vi "init_avg_scope_Qs.vi"(2 "max summed queue size (-1, unlimited)":i32) -> (8 "avg_Q_data":T1)   [LabVIEW 2023]
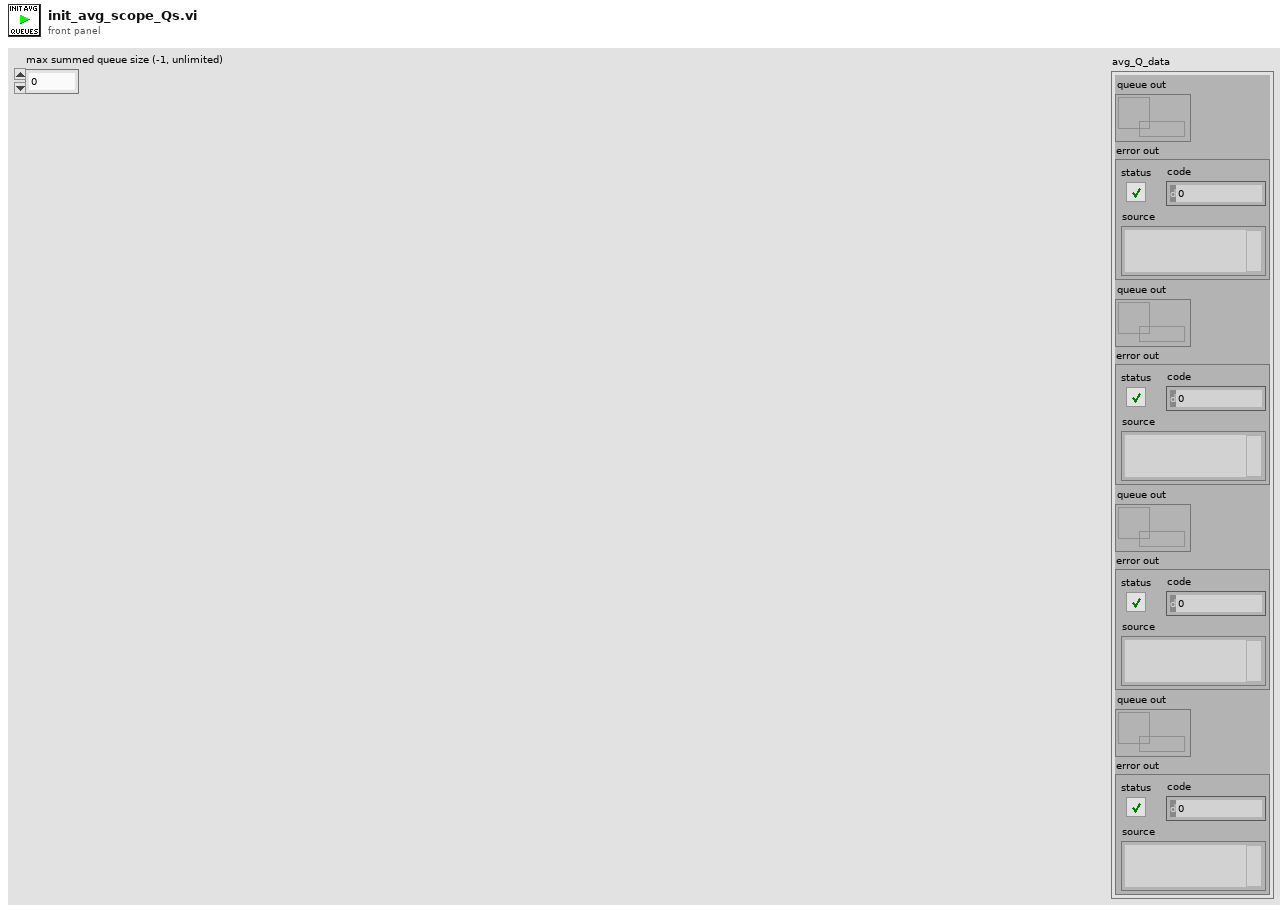
[diagram p1: front panel]
types:
  T1 = cluster{"queue out":refnum<queue>, "error out":errorcluster, "queue out":refnum<queue>, "error out":errorcluster, "queue out":refnum<queue>, "error out":errorcluster, "queue out":refnum<queue>, "error out":errorcluster}
  T2 = cluster{"wfm info":cluster{"actualSamples":i32, "absoluteInitialX":dbl, "relativeInitialX":dbl, "xIncrement":dbl, "offset":dbl, "gain":dbl, "reserved1":dbl, "reserved2":dbl}, "Offset WFm":waveform(dbl), bool}
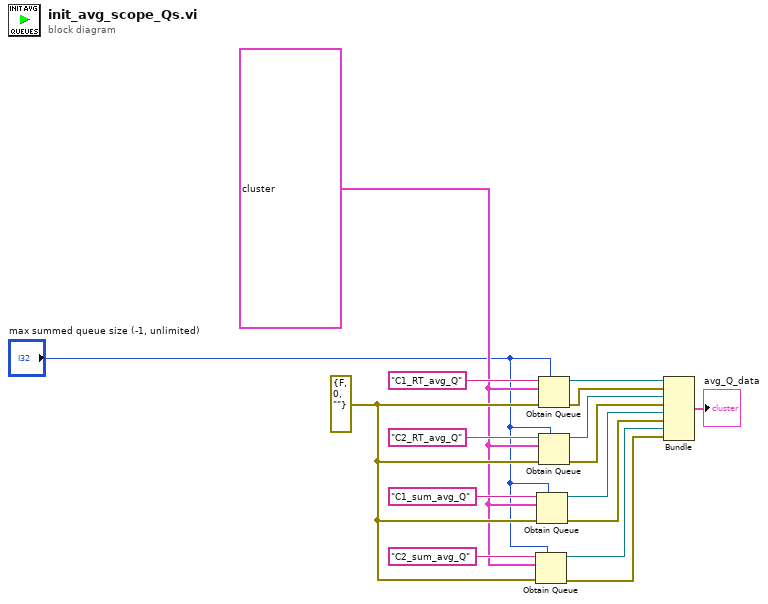
[diagram p0: block diagram]
diagram:
  w3 = T2 {"wfm info"={"actualSamples"=0, "absoluteInitialX"=0.0, "relativeInitialX"=0.0, "xIncrement"=0.0, "offset"=0.0, "gain"=0.0, "reserved1"=0.0, "reserved2"=0.0}, "Offset WFm"={"t0"=timestamp(0 s since 1904-01-01), "dt"=1.0, "Y"=[]}, FALSE} ("output cluster")
  w16 = errorcluster {"status"=FALSE, "code"=0, "source"=""} ("error in (no error)")
  n1 = Obtain Queue(max queue size (-1, unlimited)="max summed queue size (-1, unlimited)", name (unnamed)="C2_sum_avg_Q", element data type=w3, error in (no error)=w16) -> (queue out=w5:refnum<queue>, error out=w4:errorcluster)  [unwired: 1 in, 1 out]
  n2 = Obtain Queue(max queue size (-1, unlimited)="max summed queue size (-1, unlimited)", name (unnamed)="C1_sum_avg_Q", element data type=w3, error in (no error)=w16) -> (queue out=w7:refnum<queue>, error out=w6:errorcluster)  [unwired: 1 in, 1 out]
  n3 = Obtain Queue(max queue size (-1, unlimited)="max summed queue size (-1, unlimited)", name (unnamed)="C1_RT_avg_Q", element data type=w3, error in (no error)=w16) -> (queue out=w11:refnum<queue>, error out=w10:errorcluster)  [unwired: 1 in, 1 out]
  n4 = Obtain Queue(max queue size (-1, unlimited)="max summed queue size (-1, unlimited)", name (unnamed)="C2_RT_avg_Q", element data type=w3, error in (no error)=w16) -> (queue out=w9:refnum<queue>, error out=w8:errorcluster)  [unwired: 1 in, 1 out]
  n5 = Bundle("queue out"=w11, "error out"=w10, "queue out"=w9, "error out"=w8, "queue out"=w7, "error out"=w6, "queue out"=w5, "error out"=w4) -> (→"avg_Q_data":T1)  [unwired: 1 in]
